vi "Check Heartbeat.vi"(8 "error in (no error)":errorcluster, 11 "object in":refnum<class "JuPyter_Client.lvclass">) -> (0 "error out":errorcluster, 2 "Timed out/error":bool, 3 "object out":refnum<class "JuPyter_Client.lvclass">)   [LabVIEW 2018, in "JuPyter_Client.lvclass"]
doc: "Check for a live Kernel"
uses:
  JuPyter_Client.lvclass
  JuPyter_Client.lvclass/JuPyter_Client.ctl
  <vilib>/addons/zeromq/zmq_socket.lvclass
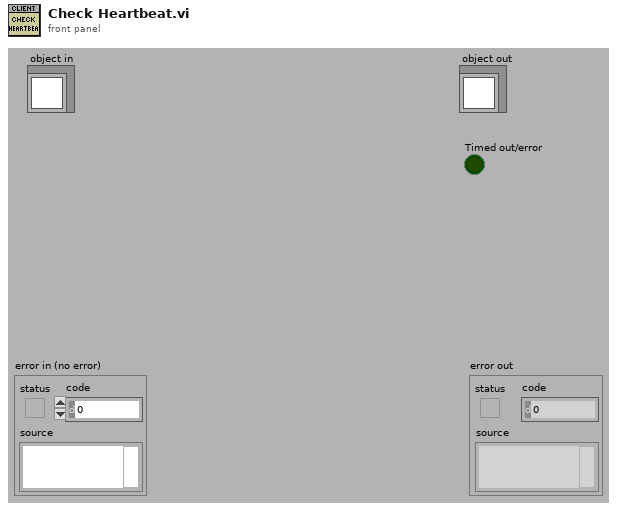
[diagram p1: front panel]
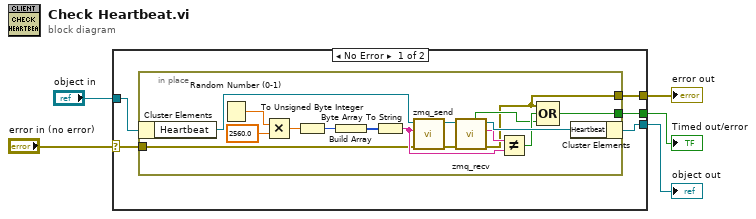
[diagram p0: block diagram]
diagram:
  n1 = case shown="No Error" "error in (no error)" {
    selector: "error in (no error)" -> [w7 w28]
    tunnel: [w8 w28] -> w3
    tunnel: [w9 w27] -> w2
    tunnel: "object in" -> [w10 w27]
    tunnel: [w6 _] -> w1
    frame No Error {
      n2 = in-place {
        in-place-border: [w11] -> w8
        in-place-border: w7 -> [w12]
        in-place-border: [w13] -> w6
        n3 = in-place-cluster #1(w10) -> ("Heartbeat"=w26:refnum<class "zmq_socket.lvclass">)
        n4 = Random Number (0-1)() -> (number: 0 to 1=w24:dbl)
        n5 = Multiply(x=w24, y=2560.0) -> (x*y=w22:dbl)
        n6 = To Unsigned Byte Integer(number=w22) -> (unsigned 8bit integer=w21:u8)
        n7 = Build Array(w21) -> (w20:u8[])
        n8 = Byte Array To String(unsigned byte array=w20) -> (string=w17:string)
        n9 = call <vilib>:"zmq_send.vi"("error in"=w12, "data"=w17, "socket in"=w26) -> ("error out"=w14:errorcluster, "socket out"=w25:refnum<class "zmq_socket.lvclass">)  [unwired: 4 in]
        n10 = call <vilib>:"zmq_recv.vi"("error in"=w14, "socket in"=w25) -> ("error out"=w11:errorcluster, "data"=w18:string, "socket out"=w19:refnum<class "zmq_socket.lvclass">, "timeout?"=w15:bool)  [unwired: 3 in, 1 out]
        n11 = Not Equal?(x=w18, y=w17) -> (x != y?=w16:bool)
        n12 = Compound Arithmetic op=OR(w11, w16, w15) -> (w13:bool)
        n13 = in-place-cluster #1("Heartbeat"=w19) -> (w9:refnum<class "JuPyter_Client.lvclass">)
      }
    }
    frame Error {
    }
  }
  "error out" <- w3
  "object out" <- w2
  "Timed out/error" <- w1
